vi "Compress Directory.vi"(8 "error in (no error)":errorcluster, 10 "archive name (root directory with .zip ending)":path, 11 "root directory (file dialog)":path) -> (0 "error out":errorcluster, 2 "archive name out":path, 3 "root directory out":path)   [LabVIEW 2020, in "Command-Line Zip.lvlib"]
uses:
  Command-Line Zip.lvlib
  <userlib>/_OpenG.lib/file/file.llb/Valid Path - Traditional__ogtk.vi
  <userlib>/_OpenG.lib/file/file.llb/Convert File Extension (Path)__ogtk.vi
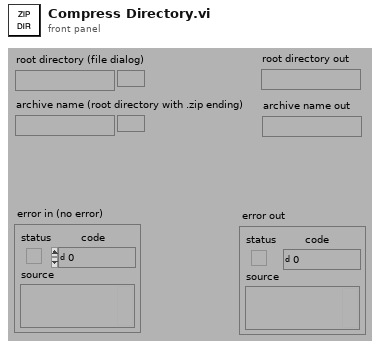
[diagram p1: front panel]
types:
  T1 = enum32{"existing file", "new file", "new or existing file", "existing dir", "new dir", "new or existing dir", "existing file (use LLBs)", "new file (use LLBs)", "new or existing file (use LLBs)", "new or existing file or directory (use LLBs)", "existing dir (use LLBs)", "new dir (use LLBs)", "new or existing dir (use LLBs)", "existing file or dir", "new file or dir", "new or existing file or dir", "existing file or dir (use LLBs)", "new file or dir (use LLBs)"}
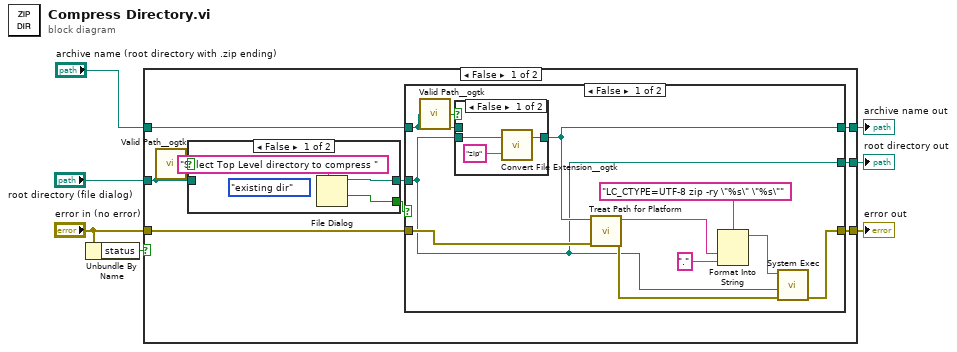
[diagram p0: block diagram]
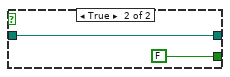
[diagram p2: hidden frame]
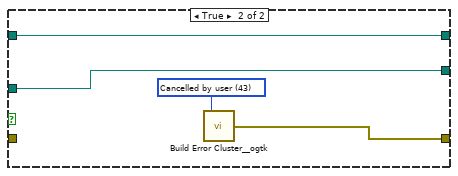
[diagram p4: hidden frame]
diagram:
  n1 = Unbundle By Name("error in (no error)") -> ("status"=w6:bool)
  n2 = case shown="False" w6 {
    tunnel: "root directory (file dialog)" -> [w13 w42]
    tunnel: "error in (no error)" -> [w11 w43]
    tunnel: [w12 w43] -> w4
    tunnel: [w10 w42] -> w3
    tunnel: [w9 w41] -> w2
    tunnel: "archive name (root directory with .zip ending)" -> [w8 w41]
    frame False {
      n3 = call-poly <userlib>:"Valid Path__ogtk.vi"("path"=w13) -> ("valid"=w14:bool)
      n4 = case shown="False" w14 {
        tunnel: [w18 w21] -> w16
        tunnel: [w17 FALSE ("cancelled")] -> w15
        tunnel: w13 -> [_ w21]
        frame False {
          (unwired) T1."existing dir" ("select mode (2)")
          n5 = File Dialog(7:"Select Top Level directory to compress " ("prompt")) -> (1:w17:bool, 3:w18:path)  [unwired: 6 in, 2 out]
        }
        frame True {
        }
      }
      n6 = case shown="False" w15 {
        tunnel: w16 -> [w23 w38]
        tunnel: w8 -> [w31 w37]
        tunnel: [w26 w40] -> w12
        tunnel: w11 -> [w25 _]
        tunnel: [w23 w38] -> w10
        tunnel: [w28 w37] -> w9
        frame False {
          n7 = call-poly <userlib>:"Valid Path__ogtk.vi"("path"=w31) -> ("valid"=w32:bool)
          n8 = case shown="False" w32 {
            tunnel: [w33 w36] -> w28
            tunnel: w23 -> [w34 _]
            tunnel: w31 -> [_ w36]
            frame False {
              n9 = call-poly <userlib>:"Convert File Extension__ogtk.vi"("new ending (none)"="zip" ("Format String"), "file name"=w34) -> ("new filename"=w33:path)  [unwired: 1 out]
            }
            frame True {
            }
          }
          n10 = call "Treat Path for Platform.vi"("error in (no error)"=w25, "File Path"=w28) -> ("error out"=w24:errorcluster, "Path for CLI"=w27:string)  [unwired: 8 in]
          n11 = Format Into String(format string="LC_CTYPE=UTF-8 zip -ry \"%s\" \"%s\"", w27, "." ("input 2")) -> (resulting string=w29:string)  [unwired: 2 in, 1 out]
          n12 = call <vilib>:"System Exec.vi"("error in (no error)"=w24, "working directory"=w23, "command line"=w29) -> ("error out"=w26:errorcluster)  [unwired: 5 in, 3 out]
        }
        frame True {
          w39 = 43 items=["No error", "Argument error", "Memory is full", "Out of zone", "End of file", "File already open", "Generic file I/O error", "File not found", "File permission error", "Disk is full", "Duplicate path", "Too many files open", "System feature not enabled", "Resource file not found", "Cannot add resource", "Resource not found", "Image not found", "Image memory error", "Pen does not exist", "Config type invalid", "Config token not found", "Config parse error", "Config memory error", "Bad external code format", "Bad external code offset", "External code not present", "Null window", "Destroy window error", "Null menu", "Print aborted", "Bad print record", "Print driver error", "Windows error during printing", "Memory error during printing", "Print dialog error", "Generic print error", "Invalid device refnum", "Device not found", "Device parameter error", "Device unit error", "Cannot open device", "Device call aborted", "Generic error", "Cancelled by user", "Object ID too low", "Object ID too high", "Object not in heap", "Unknown heap", "Unknown object (invalid DefProc)", "Unknown object (DefProc not in table)", "Message out of range", "Invalid (null) method", "Unknown message", "Manager call not supported", "Bad address", "Network operation in progress", "Network operation timed out", "Connection is busy", "Network attribute not supported", "Network error", "Address in use", "System out of memory", "Connection aborted", "Connection refused", "Not connected", "Already connected", "Connection closed", "Initialization error (interapplication manager)", "Bad occurrence", "Wait on unbound occurrence handler", "Occurrence queue overflow", "Datalog type conflict", "Unused", "Unrecognized type (interapplication manager)", "Memory corrupt", "Failed to make temporary DLL", "Old CIN version", "Drag socket not found", "Failed to load drop-object", "Failed to register OLE object", "Failed to release OLE object", "Format specifier type mismatch", "Unknown format specifier", "Too few format specifiers", "Too many format specifiers", "Scan failed", "Newer CIN version", "Error converting to variant", "Runtime menu error", "Password tampered", "Variant attribute not found", "Incompatible variant data type", "Event data is not available", "Event Store is not present", "Occurrence is not found", "Event Queue is not created", "Event info is not available", "Refnum passed is NULL", "Error retrieving Class GUID", "Error retrieving CoClass GUID", "Error retrieving TypeLib GUID.", "Bad built application magic bytes.", "Specific driver is different from the specific driver associated with the Logical Name.", "There is no session opened to the class driver.", "Max Error", "MAX - Error with config objects", "MAX - Error loading configuration", "MAX - Group not supported"]
          n13 = call <userlib>:"Build Error Cluster__ogtk.vi"("code"=w39) -> ("error out"=w40:errorcluster)  [unwired: 1 in]
        }
      }
    }
    frame True {
    }
  }
  "error out" <- w4
  "root directory out" <- w3
  "archive name out" <- w2
